vi "b030查询是否有产品ID.vi"(8 "error in (no error)":errorcluster, 11 "转向器总成ID":string) -> (0 "error out":errorcluster, 3 "无重号":bool)   [LabVIEW 2013]
uses:
  <vilib>/Utility/error.llb/whitespace.ctl
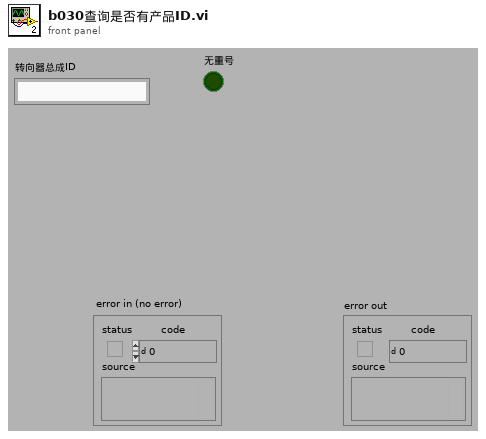
[diagram p1: front panel]
types:
  T1 = typedef "whitespace.ctl" = u16
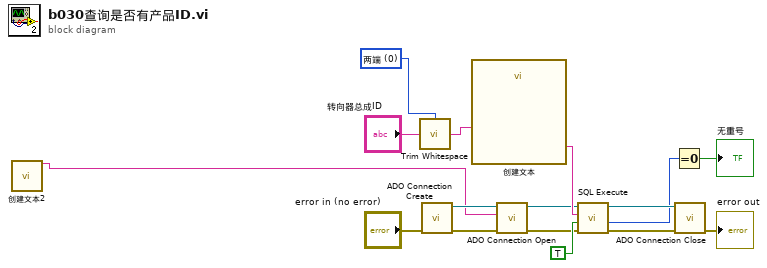
[diagram p0: block diagram]
diagram:
  w13 = T1 0 items=["两端", "字符串首端", "字符串末端"] ("location (both)")
  n1 = call "创建文本2"() -> ("Result"=w1:string)  [unwired: 14 in, 1 out]
  n2 = call <vilib>:"Trim Whitespace.vi"("string"="转向器总成ID", "location (both)"=w13) -> ("trimmed string"=w2:string)
  n3 = call "ADO Connection Create.vi"("error in (no error)"="error in (no error)") -> ("error out"=w15:errorcluster, "ADODB._Connection Out"=w16:refnum<k7>)  [unwired: 9 out]
  n4 = call "创建文本"("产品ID"=w2) -> ("Result"=w9:string)  [unwired: 13 in, 1 out]
  n5 = call "ADO Connection Open.vi"("error in (no error)"=w15, "ConnectionString"=w1, "ADODB._Connection In"=w16) -> ("error out"=w7:errorcluster, "ADODB._Connection Out"=w8:refnum<k7>)  [unwired: 7 out]
  n6 = call "SQL Execute.vi"("error in (no error)"=w7, "Return Data (T)"=TRUE, "Command Text"=w9, "ADODB._Connection In"=w8) -> ("error out"=w5:errorcluster, "Rows Fetched"=w4:i32, "ADODB._Connection Out"=w6:refnum<k7>)  [unwired: 4 in, 1 out]
  n7 = Equal To 0?(x=w4) -> (x = 0?=→"无重号":bool)
  n8 = call "ADO Connection Close.vi"("error in (no error)"=w5, "ADODB._Connection In"=w6) -> ("error out"=→"error out":errorcluster)  [unwired: 9 out]
